vi "Man_Power_List.vi"(6 "Man Power Ref":refnum<vi>, 8 "error in (no error)":errorcluster, 11 "Ref in":T3={"MS SQL Connection"=refnum, "UDL File"=path "", "Time"="", "DCODE"="", "WIP+1"=0, "MC No?"=0, "POKAYOKE?"=FALSE, "Expected Result"="", "Result [Status]"="", "Clock"=0.0, "RFID"="", "WIP Queue"=refnum, "TS Parameter"={"ProfitCenterCode"="", "LineCode"="", "WorkOrderNumber"="", "Model"="", "Model_with_Prefix"="", "VendorCode"="", "SetParameterDateCode"="", "PokaYoke"=0, "Target"=1, "Live_DateCode"="", "CustomerPartNumber"="", "Hand"="", "sBarcode"=FALSE, "FCA"=0, "Ent_Stamp"=timestamp(0 s since 1904-01-01), "STS_CD"=0.0}, "Data_Queue"=[], "RFID Serial No."=""} {"TS Parameter"."FCA" format="%01d"; "TS Parameter"."Target" min=1 max=100000; "TS Parameter"."PokaYoke" min=0 max=1}) -> (0 "error out":errorcluster, 4 "Man Power":T1)   [LabVIEW 2020]
uses:
  Controls/TD SQL.ctl
  <vilib>/addons/database/Connection.llb/Conn ObjectReference.ctl
  Controls/WIP_State.ctl
  Controls/TS_Parameter.ctl
  Controls/Man_Power.ctl
  Controls/Line Man Power.ctl
  <vilib>/addons/database/_DB Variant To Data/Database Variant To Data.xnode
  <vilib>/addons/database/NI_Database_API.lvlib
panel:
  in  "OP10":T2={"Clock No."="21603", "Name"="Devaseelan"}
  # "Clock No."
  # "Operator Name"
  # "Clock No."
  # "Operator Name"
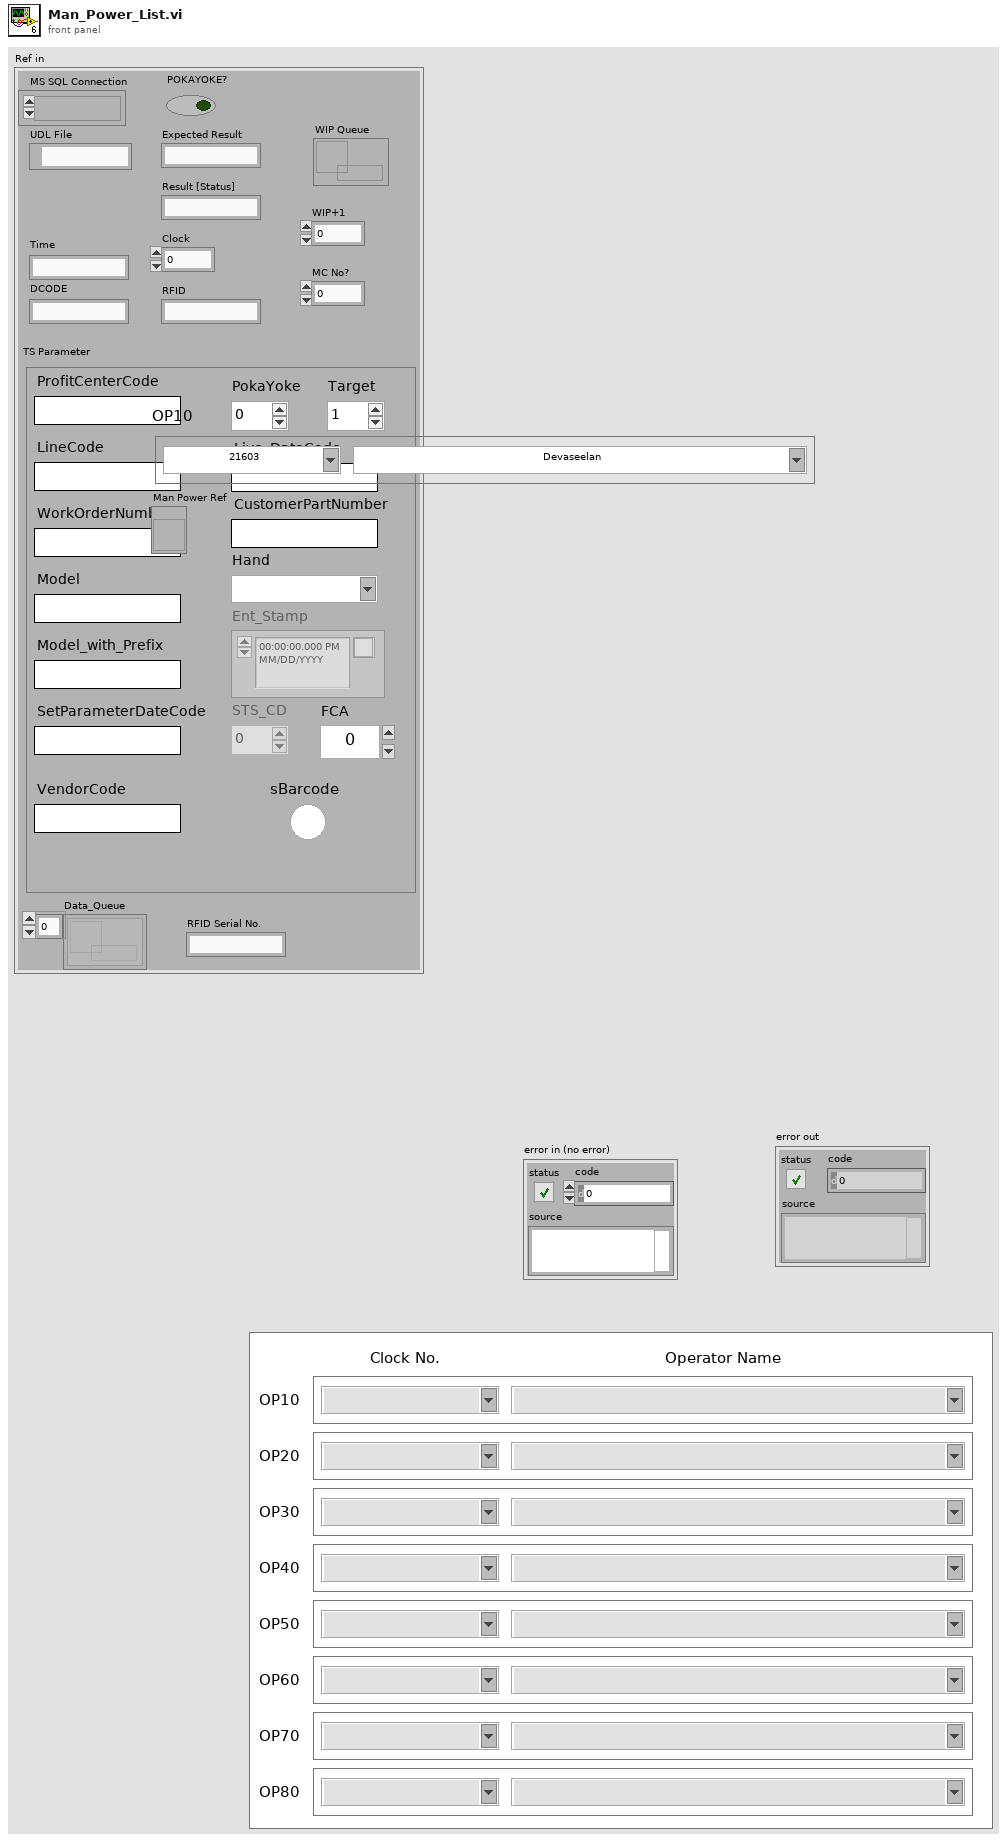
[diagram p1: front panel]
types:
  T1 = typedef "Line Man Power.ctl" = cluster{"OP10":T2, "OP20":T2, "OP30":T2, "OP40":T2, "OP50":T2, "OP60":T2, "OP70":T2, "OP80":T2}
  T2 = typedef "Man_Power.ctl" = cluster{"Clock No.":string, "Name":string}
  T3 = typedef "TD SQL.ctl" = cluster{"MS SQL Connection":T4, "UDL File":path, "Time":string, "DCODE":string, "WIP+1":i64, "MC No?":i32, "POKAYOKE?":bool, "Expected Result":string, "Result [Status]":string, "Clock":dbl, "RFID":string, "WIP Queue":refnum<queue>, "TS Parameter":T5, "Data_Queue":refnum<queue>[], "RFID Serial No.":string}
  T4 = typedef "NI_Database_API.lvlib/Conn ObjectReference.ctl" = refnum<k1>
  T5 = typedef "TS_Parameter.ctl" = cluster{"ProfitCenterCode":string, "LineCode":string, "WorkOrderNumber":string, "Model":string, "Model_with_Prefix":string, "VendorCode":string, "SetParameterDateCode":string, "PokaYoke":i32, "Target":i32, "Live_DateCode":string, "CustomerPartNumber":string, "Hand":string, "sBarcode":bool, "FCA":i32, "Ent_Stamp":timestamp, "STS_CD":dbl}
  T6 = cluster{"[0]":T2, "[1]":T2, "[2]":T2, "[3]":T2, "[4]":T2, "[5]":T2, "[6]":T2, "[7]":T2}
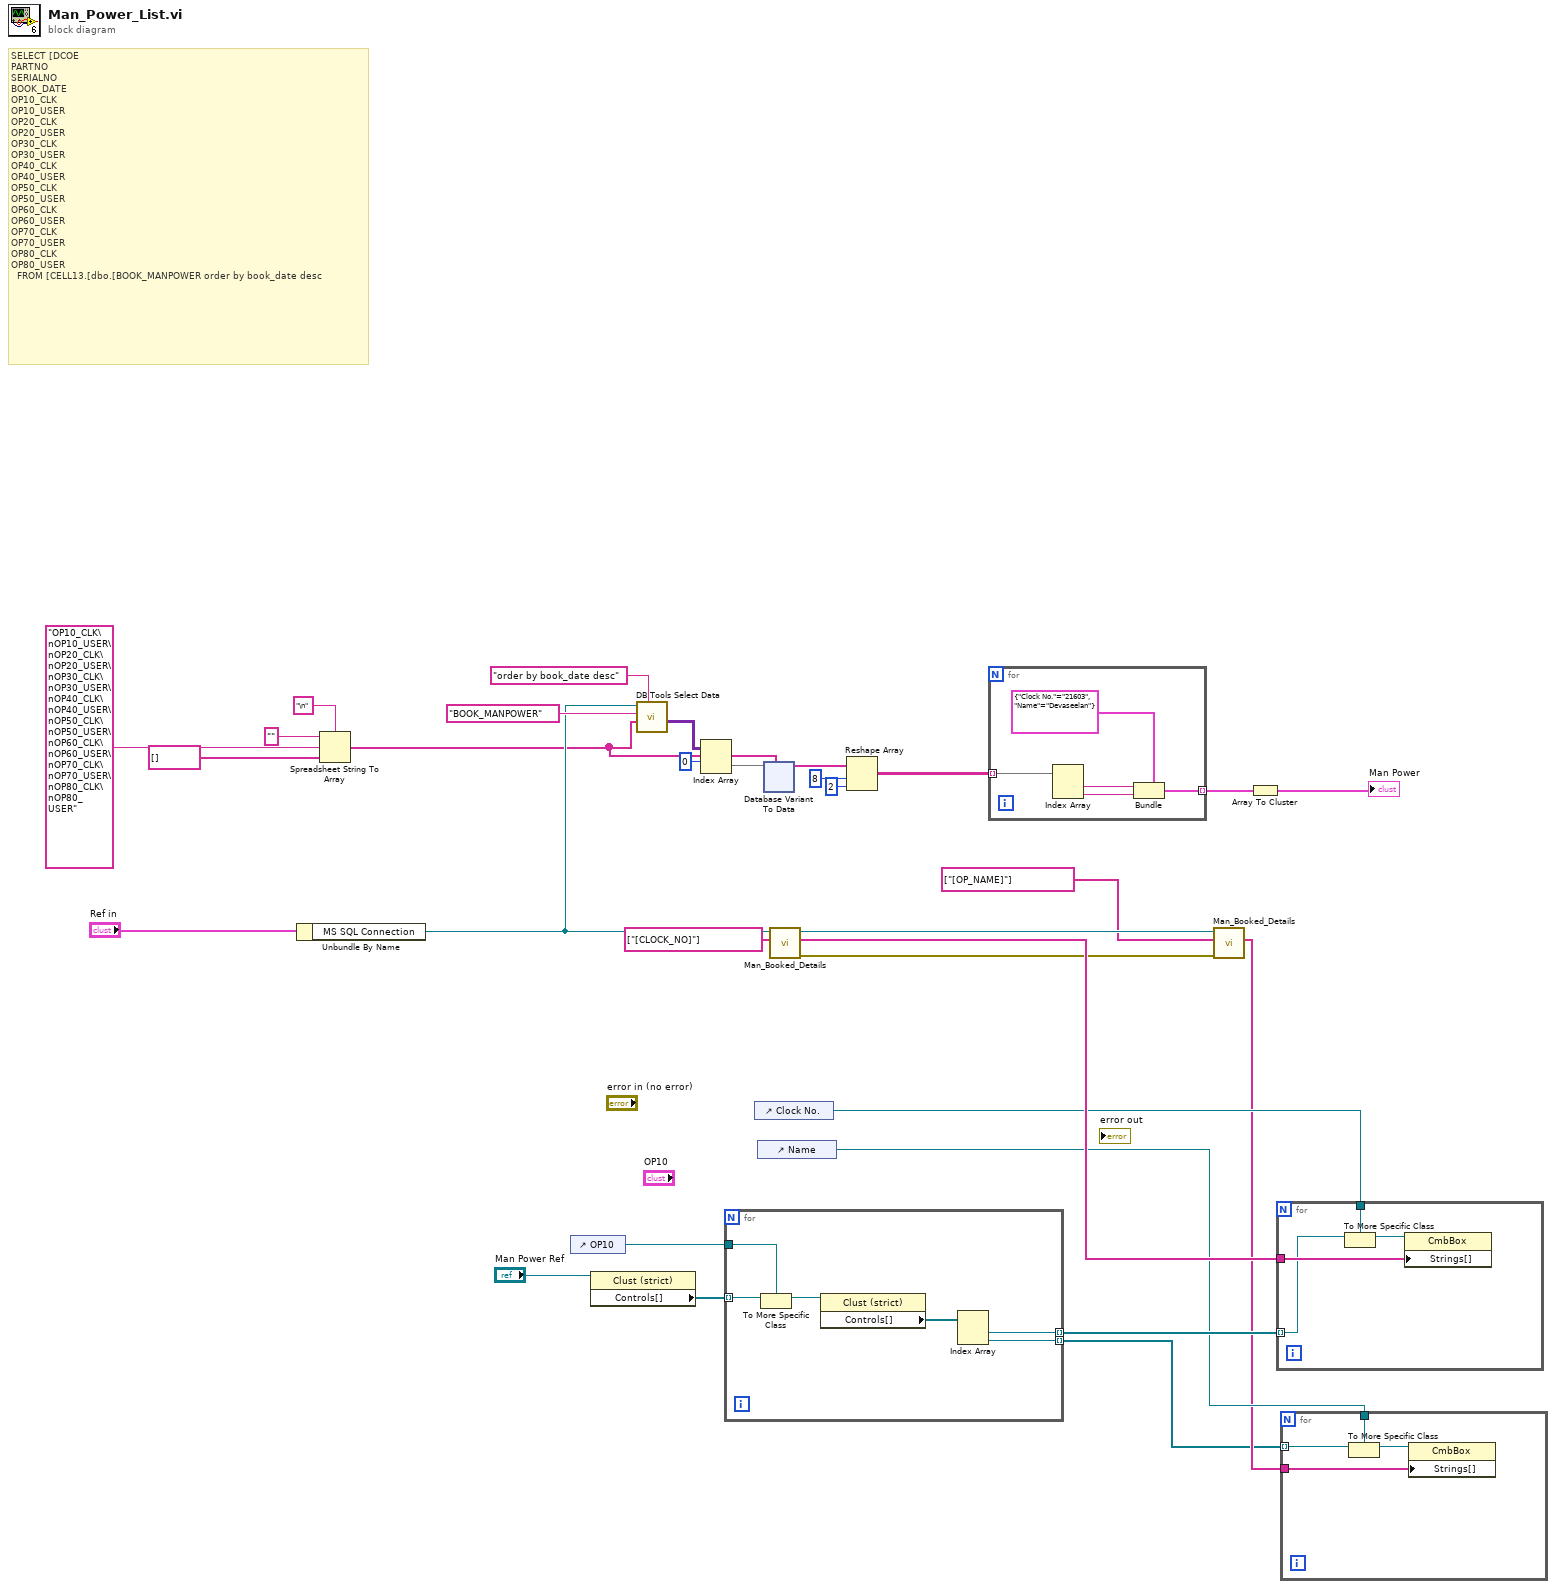
[diagram p0: block diagram]
diagram:
  # "SELECT [DCOE\nPARTNO\nSERIALNO\nBOOK_DATE\nOP10_CLK\nOP10_USER\nOP20_CLK\nOP20_USER\nOP30_CLK\nOP30_USER\nOP40_CLK\nOP40_USER\nOP50_CLK\nOP50_USER\nOP60_CLK\nOP60_USER\nOP70_CLK\nOP70_USER\nOP80_CLK\nOP80_USER\n  FROM [CELL13.[dbo.[BOOK_MANPOWER order by book_date desc"
  n1 = Unbundle By Name("Ref in") -> ("MS SQL Connection"=w17:T4)
  n2 = Spreadsheet String To Array(delimiter (Tab)="\n", format string="" ("table"), spreadsheet string="OP10_CLK\nOP10_USER\nOP20_CLK\nOP20_USER\nOP30_CLK\nOP30_USER\nOP40_CLK\nOP40_USER\nOP50_CLK\nOP50_USER\nOP60_CLK\nOP60_USER\nOP70_CLK\nOP70_USER\nOP80_CLK\nOP80_USER" ("table"), array type (2D Dbl)=string[] []) -> (array=w8:string[])
  n3 = control-ref of="OP10"() -> (w28:refnum<vi>)
  n4 = property class="Clust (strict)"(reference="Man Power Ref") -> ("Controls[]"=w29:refnum<vi>[])  [unwired: 1 in, 2 out]
  n5 = call <vilib>:"DB Tools Select Data.vi"("condition"="order by book_date desc", "columns"=w8, "table"="BOOK_MANPOWER", "connection reference"=w17) -> ("data"=w14:variant[][])  [unwired: 2 in, 2 out]
  n6 = Index Array(array=w14, index (row)=0) -> (element=w9:variant[])  [unwired: 1 in]
  n7 = for {
    tunnel: w29 -> [w37] mode=indexing
    tunnel: w28 -> [w35]
    tunnel: [w33] -> w27 mode=indexing
    tunnel: [w32] -> w20 mode=indexing
    n8 = To More Specific Class(target class=w35, reference=w37) -> (specific class reference=w36:refnum<vi>)  [unwired: 1 in, 1 out]
    n9 = property class="Clust (strict)"(reference=w36) -> ("Controls[]"=w34:refnum<vi>[])  [unwired: 1 in, 2 out]
    n10 = Index Array(array=w34) -> (element #1=w33:refnum<vi>, element #2=w32:refnum<vi>)  [unwired: 2 in]
  }
  n11 = control-ref of="Clock No."() -> (w26:refnum<vi>)
  n12 = control-ref of="Name"() -> (w22:refnum<vi>)
  n13 = xnode "Database Variant To Data"("database variant"=w9, "type"=w8) -> ("data"=w7:string[])  [unwired: 1 in, 1 out]
  n14 = call "Man_Booked_Details.vi"("Column"=string[] ["[CLOCK_NO]"] ("array"), "Refnum in"=w17) -> ("error out"=w24:errorcluster, "Data"=w30:string[], "Refnum Out"=w25:T4)  [unwired: 7 in]
  n15 = Reshape Array(w7, 8 ("dimension size"), 2 ("dimension size")) -> (w4:string[][])
  n16 = for {
    tunnel: w4 -> [w42] mode=indexing
    tunnel: [w38] -> w3 mode=indexing
    n17 = Index Array(array=w42) -> (element #1=w40:string, element #2=w39:string)  [unwired: 2 in]
    n18 = Bundle(cluster=T2 {"Clock No."="21603", "Name"="Devaseelan"} ("OP10"), "Clock No."=w40, "Name"=w39) -> (w38:T2)
  }
  n19 = call "Man_Booked_Details.vi"("error in (no error)"=w24, "Column"=string[] ["[OP_NAME]"] ("array"), "Refnum in"=w25) -> ("Data"=w21:string[])  [unwired: 6 in, 2 out]
  n20 = Array To Cluster(array=w3) -> (cluster=→"Man Power":T6)
  n21 = for {
    tunnel: w30 -> [w46]
    tunnel: w27 -> [w45] mode=indexing
    tunnel: w26 -> [w43]
    n22 = To More Specific Class(target class=w43, reference=w45) -> (specific class reference=w44:refnum<vi>)  [unwired: 1 in, 1 out]
    n23 = property class="CmbBox"(reference=w44, "Strings[]"=w46) -> ()  [unwired: 1 in, 2 out]
  }
  n24 = for {
    tunnel: w21 -> [w50]
    tunnel: w20 -> [w49] mode=indexing
    tunnel: w22 -> [w47]
    n25 = To More Specific Class(target class=w47, reference=w49) -> (specific class reference=w48:refnum<vi>)  [unwired: 1 in, 1 out]
    n26 = property class="CmbBox"(reference=w48, "Strings[]"=w50) -> ()  [unwired: 1 in, 2 out]
  }
